vi "DAQ module.vi"(8 "error in (no error)":errorcluster) -> (0 "error out":errorcluster)   [LabVIEW 2016]
uses:
  Controls/Gain modes.ctl
  General/Controls/Queue modes.ctl
  General/Controls/staus modes.ctl
  General/Controls/DAQ device list.ctl
  General/Controls/data modes.ctl
  <vilib>/DAQmx/read.llb/DAQmx Read (Analog DBL 1Chan 1Samp).vi
  <vilib>/DAQmx/miscellaneous.llb/DAQmx Fill In Error Info.vi
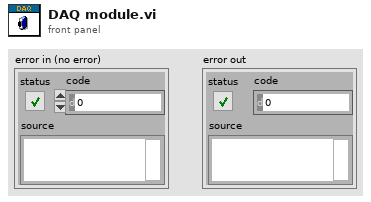
[diagram p1: front panel]
types:
  T1 = cluster{"seconds since 1Jan1904":timestamp, "Numeric 2":dbl}[]
  T2 = typedef "Queue modes.ctl" = enum16{"Initialise", "Destroy", "Get"}
  T3 = typedef "Gain modes.ctl" = enum16{"Initalise", "Get", "Set"}
  T4 = typedef "References.ctl" = cluster{"Tab Control":refnum<vi>, "Logo 1":refnum<vi>, "Logo 2":refnum<vi>, "Connect Actuator":refnum<vi>, "LIVE DATA":refnum<vi>, "Speed":refnum<vi>, "Home position":refnum<vi>, "Limit position":refnum<vi>, "Trigger":refnum<vi>, "Current position":refnum<vi>, "Connect Camera":refnum<vi>, "TEST DATA":refnum<vi>, "LIVE DATA Force":refnum<vi>, "Connect DAQ":refnum<vi>, "Initialised":refnum<vi>, "Test":refnum<vi>}
  T5 = typedef "staus modes.ctl" = enum16{"Status", "Testing", "Webcam", "DAQ", "Actuator", "Initialise"}
  T6 = typedef "DAQ device list.ctl" = enum16{"USB-6211", "NI myDAQ", "NI 9211"}
  T7 = typedef "data modes.ctl" = enum16{"Initalise", "Status", "Process", "Add load", "Add position"}
  T8 = enum16{"open", "replace", "create", "open or create", "replace or create", "replace or create with confirmation"}
  T9 = cluster{"seconds since 1Jan1904":timestamp, "data":dbl}[]
  T10 = typedef "DAQ queue.ctl" = cluster{"Sate":T11, "Data":variant}
  T11 = typedef "Queue states.ctl" = enum16{"Shutdown", "Save data", "Record", "Read", "Setup", "Zero", "Connect", "Initialise"}
  T12 = typedef "UEs.ctl" = cluster{"Read position":refnum<user-event>, "Check home":refnum<user-event>, "Record":refnum<user-event>, "Abort controller":refnum<user-event>, "Remote test":refnum<user-event>, "Test setup":refnum<user-event>, "Conditional wait":refnum<user-event>, "Abort move":refnum<user-event>, "Wait done":refnum<user-event>, "Send trigger":refnum<user-event>, "Initalising":refnum<user-event>, "Initalisation complete":refnum<user-event>}
  T13 = cluster{"seconds since 1Jan1904":timestamp, "Numeric":dbl}
  T14 = cluster{"seconds since 1Jan1904":timestamp, "Numeric":dbl}[]
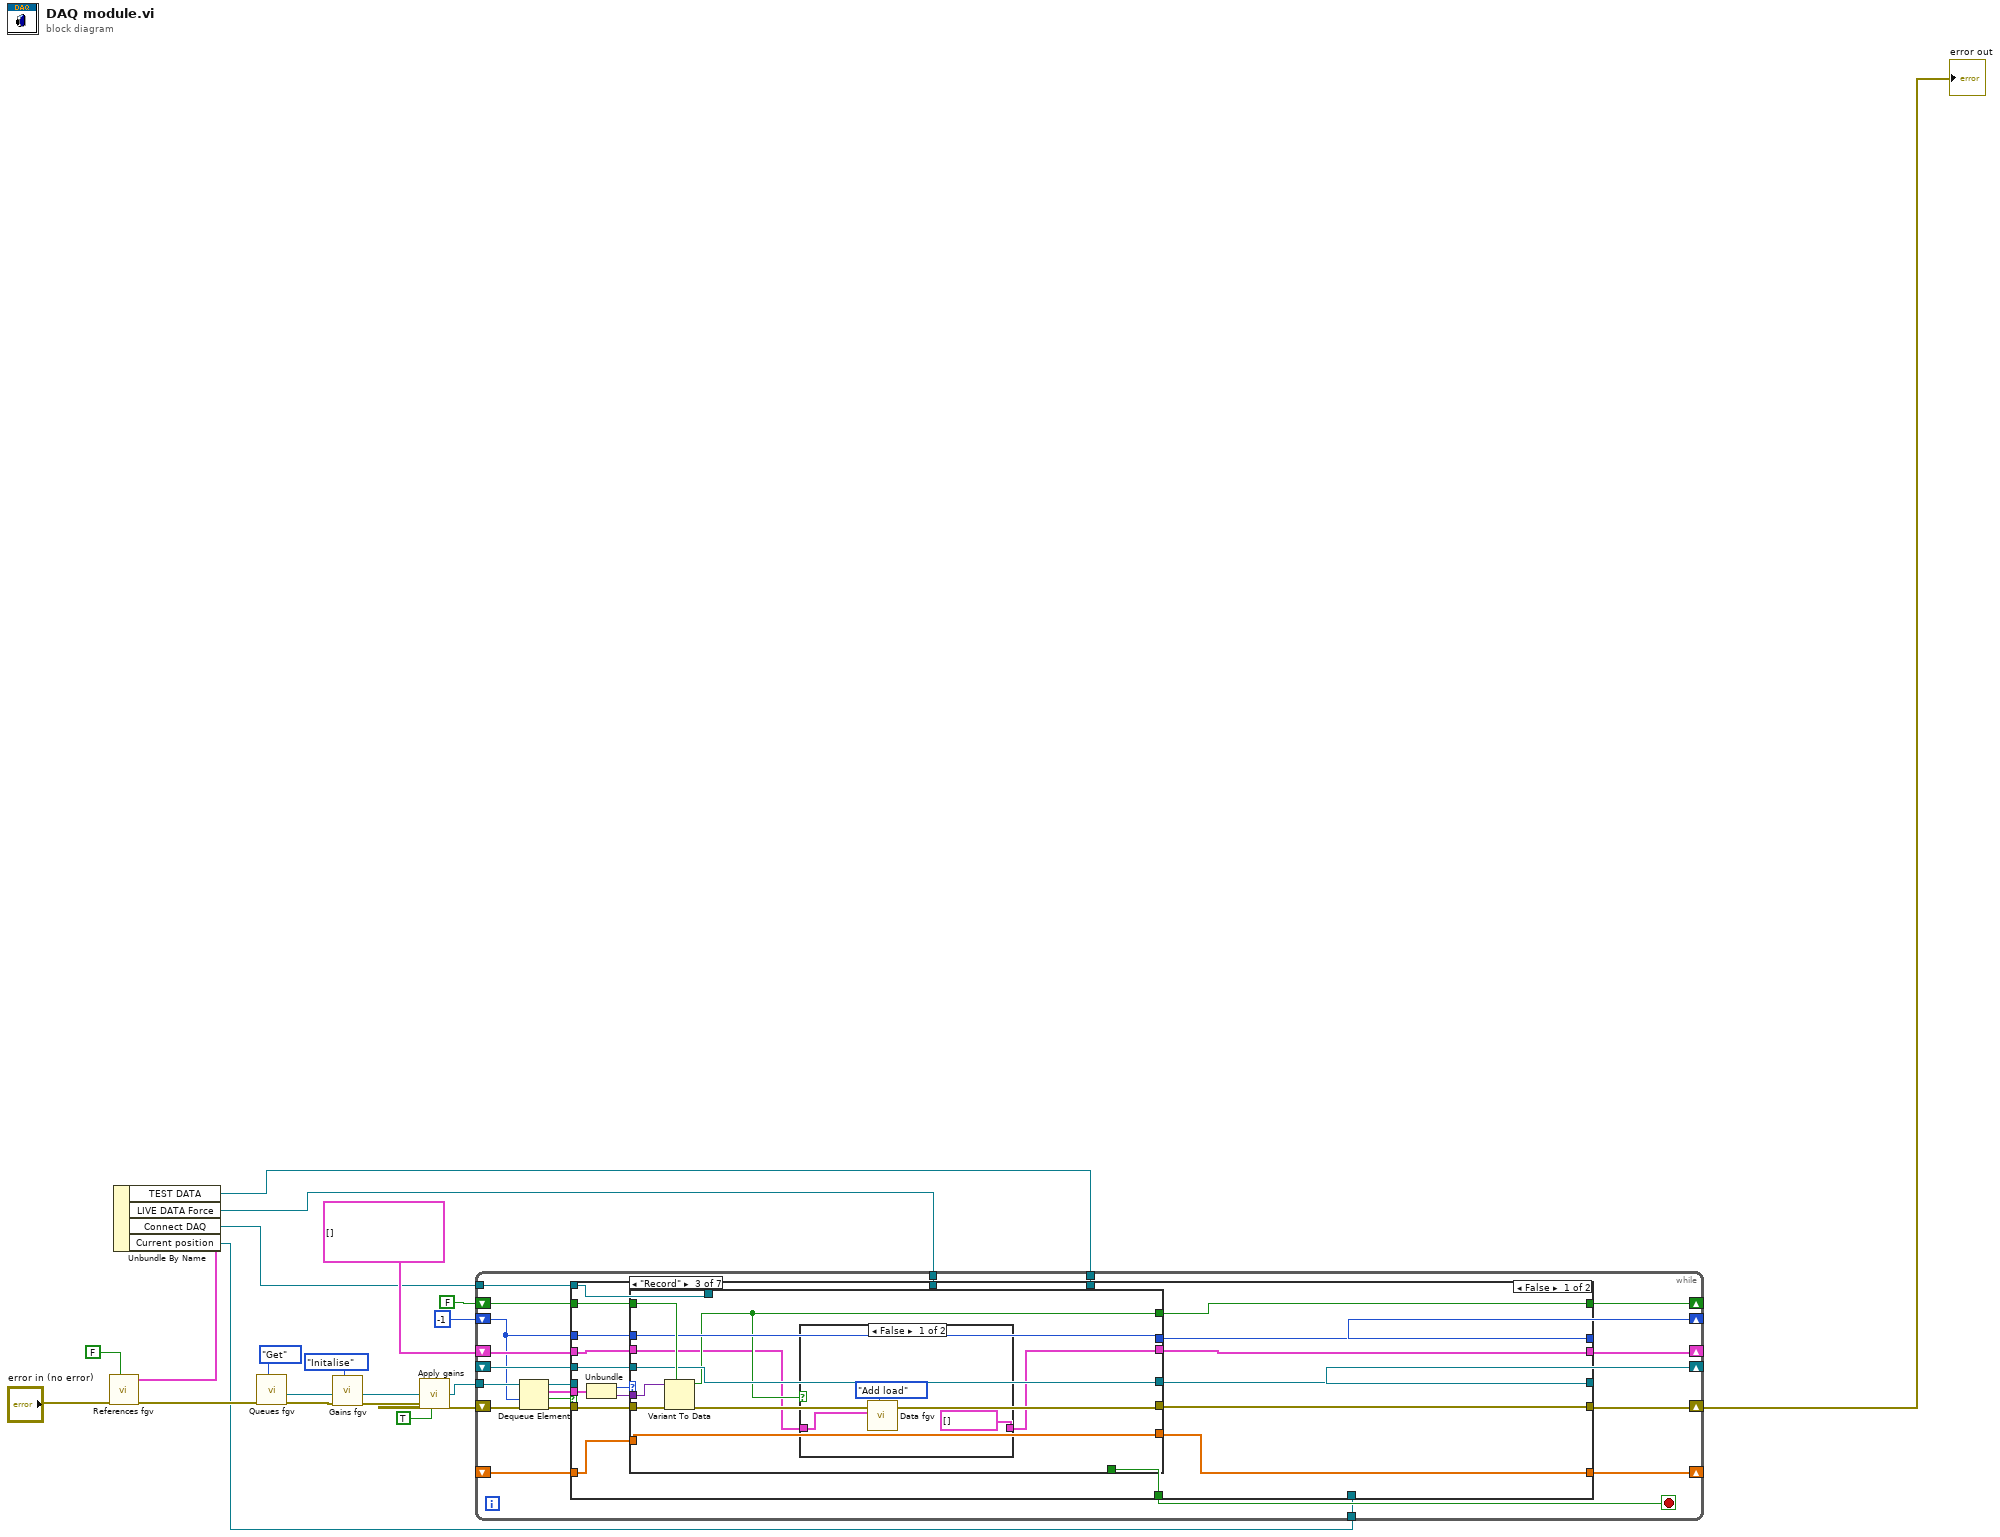
[diagram p0: block diagram]
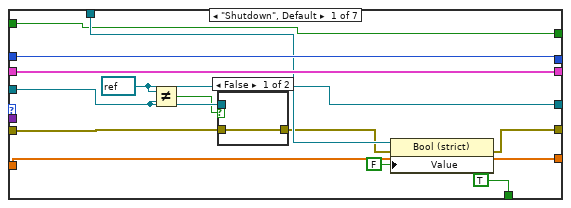
[diagram p2: hidden frame]
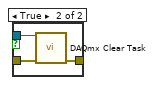
[diagram p3: hidden frame]
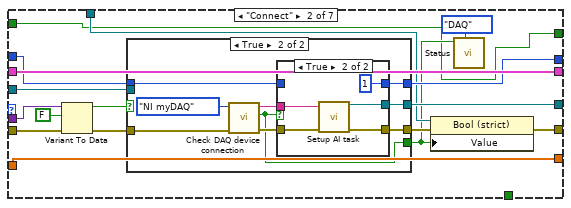
[diagram p4: hidden frame]
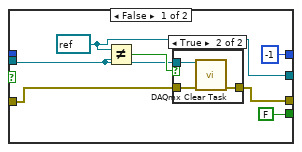
[diagram p5: hidden frame]
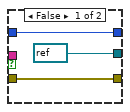
[diagram p7: hidden frame]
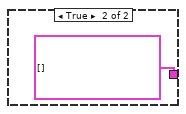
[diagram p8: hidden frame]
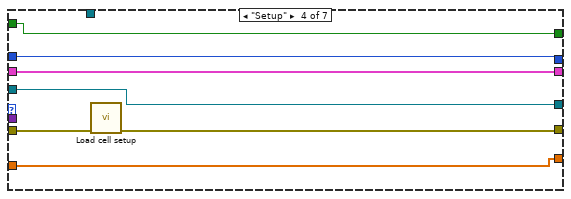
[diagram p9: hidden frame]
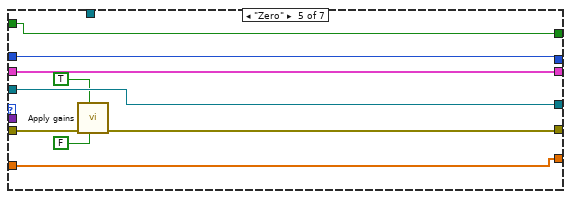
[diagram p10: hidden frame]
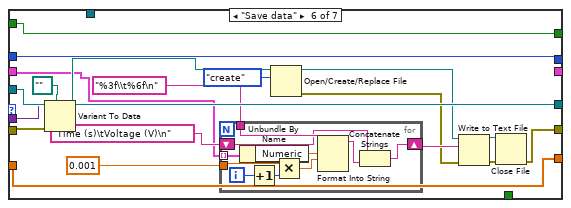
[diagram p11: hidden frame]
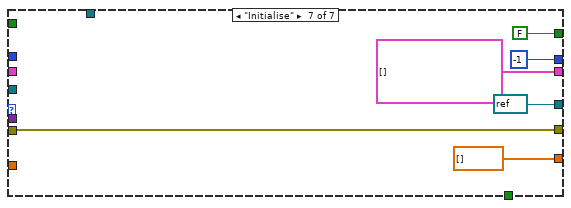
[diagram p12: hidden frame]
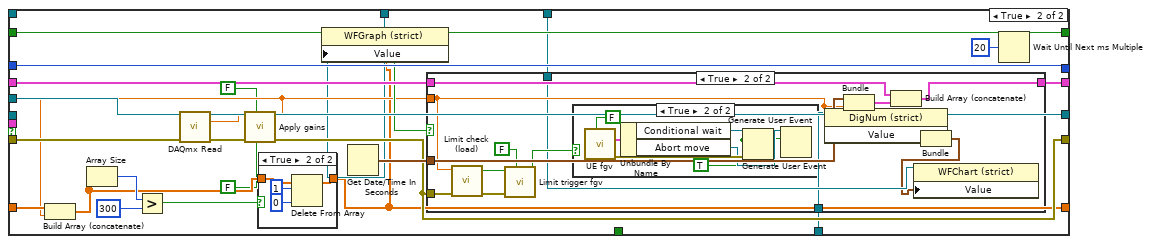
[diagram p13: hidden frame]
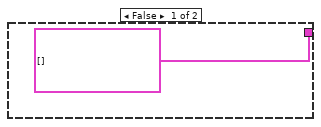
[diagram p14: hidden frame]
diagram:
  n1 = call "References fgv.vi"("Set?"=FALSE, "error in (no error)"="error in (no error)") -> ("error out"=w8:errorcluster, "Cluster"=w5:T4)  [unwired: 8 in]
  n2 = Unbundle By Name(w5) -> ("TEST DATA"=w2:refnum<vi>, "LIVE DATA Force"=w3:refnum<vi>, "Connect DAQ"=w4:refnum<vi>, "Current position"=w1:refnum<vi>)
  n3 = call "Queues fgv.vi"("Modes"=Queue_modes."Get", "error in (no error)"=w8) -> ("error in (no error) 2"=w18:errorcluster, "DAQ"=w17:refnum<queue>)  [unwired: 6 in, 2 out]
  n4 = call "Gains fgv.vi"("Mode"=Gain_modes."Initalise", "error in (no error)"=w18) -> ("error out"=w14:errorcluster)  [unwired: 7 in, 2 out]
  n5 = call "Apply gains.vi"("Initalise"=TRUE, "error in (no error)"=w14) -> ("error out"=w12:errorcluster)  [unwired: 8 in, 1 out]
  n6 = while {
    shift-right: [w40] -> _
    shift-left: _ -> [w41]
    shift-right: [w39] -> w10
    shift-left: w12 -> [w33]
    shift-right: [w38] -> _
    shift-left: T1 [] -> [w37]
    tunnel: w17 -> [w36]
    shift-right: [w29] -> _
    shift-left: -1 ("timeout in ms (-1)") -> [w30]
    tunnel: w4 -> [w28]
    shift-right: [w26] -> _
    shift-left: FALSE -> [w27]
    shift-right: [w23] -> _
    shift-left: _ -> [w24]
    tunnel: w3 -> [w22]
    tunnel: w2 -> [w21]
    tunnel: w1 -> [w20]
    stop <- w25 stop-if-true
    n7 = Dequeue Element(queue=w36, timeout in ms (-1)=w30, error in (no error)=w33) -> (queue out=w35:refnum<queue>, element=w31:T10, timed out?=w32:bool, error out=w34:errorcluster)
    n8 = case shown="False" w32 {
      tunnel: w41 -> [w50 w209]
      tunnel: w34 -> [w55 w203]
      tunnel: [w53 w208] -> w40
      tunnel: [w54 w190] -> w39
      tunnel: [w51 w207] -> w38
      tunnel: w37 -> [w52 w206]
      tunnel: w35 -> [_ _]
      tunnel: w31 -> [w58 _]
      tunnel: w30 -> [w49 w205]
      tunnel: [w48 w205] -> w29
      tunnel: w28 -> [w47 _]
      tunnel: w27 -> [w46 w204]
      tunnel: [w45 w204] -> w26
      tunnel: [w44 _] -> w25
      tunnel: w24 -> [w42 w200]
      tunnel: [w43 w188] -> w23
      tunnel: w22 -> [_ w189]
      tunnel: w21 -> [_ w187]
      tunnel: w20 -> [_ w186]
      frame False {
        n9 = Unbundle(w58) -> ("Sate"=w57:T11, "Data"=w56:variant)
        n10 = case shown="\"Record\"" w57 {
          tunnel: w56 -> [_ w87 w129 _ _ w164 _]
          tunnel: w55 -> [w70 w88 w130 w138 w145 w166 w183]
          tunnel: [w62 w81 w127 w137 w144 w153 w183] -> w54
          tunnel: [w69 w92 w126 w136 w147 w167 refnum<k21> refnum ("task out")] -> w53
          tunnel: w52 -> [w71 w91 w123 w139 w148 w152 _]
          tunnel: [w71 w91 w122 w139 w148 _ T9 []] -> w51
          tunnel: w50 -> [w68 w83 w126 w136 w147 w167 _]
          tunnel: w49 -> [w66 w90 w125 w140 w149 w169 _]
          tunnel: [w66 w89 w125 w140 w149 w169 -1 ("timeout in ms (-1)")] -> w48
          tunnel: w47 -> [w65 w80 _ _ _ _ _]
          tunnel: w46 -> [w61 w77 w128 w141 w150 w168 _]
          tunnel: [w61 w77 w124 w141 w150 w168 FALSE] -> w45
          tunnel: [TRUE _ _ _ _ _ _] -> w44
          tunnel: [w59 w76 w121 w135 w146 w151 dbl[] []] -> w43
          tunnel: w42 -> [w59 w76 w121 w135 w146 w151 _]
          frame "Shutdown", Default {
            w69 = refnum<k21> refnum ("task out")
            n11 = Not Equal?(x=w69, y=w68) -> (x != y?=w67:bool)
            n12 = case shown="False" w67 {
              tunnel: w70 -> [w72 w75]
              tunnel: [w72 w74] -> w63
              tunnel: w68 -> [_ w73]
              frame False {
              }
              frame True {
                n13 = call <vilib>:"DAQmx Clear Task.vi"("task in"=w73, "error in"=w75) -> ("error out"=w74:errorcluster)  [unwired: 13 in]
              }
            }
            n14 = property class="Bool (strict)"(reference=w65, error in=w63, "Value"=FALSE) -> (error out=w62:errorcluster)  [unwired: 1 out]
          }
          frame "Connect" {
            n15 = Variant To Data(error in=w88, type=FALSE, Variant=w87) -> (data=w84:bool, error out=w86:errorcluster)
            n16 = case shown="True" w84 {
              tunnel: [w95 w109] -> w82
              tunnel: [w97 w108] -> w92
              tunnel: w90 -> [_ w107]
              tunnel: [-1 ("timeout in ms (-1)") w106] -> w89
              tunnel: w86 -> [w94 w105]
              tunnel: w83 -> [w98 _]
              tunnel: [FALSE ("x != y?") w104] -> w78
              frame False {
                w97 = refnum<k21> refnum ("task out")
                n17 = Not Equal?(x=w97, y=w98) -> (x != y?=w99:bool)
                n18 = case shown="True" w99 {
                  tunnel: w94 -> [w100 w103]
                  tunnel: [w100 w102] -> w95
                  tunnel: w98 -> [_ w101]
                  frame False {
                  }
                  frame True {
                    n19 = call <vilib>:"DAQmx Clear Task.vi"("task in"=w101, "error in"=w103) -> ("error out"=w102:errorcluster)  [unwired: 13 in]
                  }
                }
              }
              frame True {
                n20 = call "Check DAQ device connection.vi"("error in (no error)"=w105, "DAQ Device"=DAQ_device_list."NI myDAQ") -> ("error out"=w111:errorcluster, "Device Present?"=w104:bool, "DAQmx Device Name"=w112:tag)  [unwired: 7 in]
                n21 = case shown="True" w104 {
                  tunnel: w111 -> [w114 w120]
                  tunnel: w112 -> [_ w119]
                  tunnel: [refnum<k21> refnum ("task out") w118] -> w108
                  tunnel: [w114 w117] -> w109
                  tunnel: w107 -> [w113 _]
                  tunnel: [w113 1 ("timeout in ms (-1)")] -> w106
                  frame False {
                  }
                  frame True {
                    n22 = call "Setup AI task.vi"("error in"=w120, "DAQmx Device Name"=w119) -> ("error out"=w117:errorcluster, "task out"=w118:refnum<k21>)  [unwired: 8 in]
                  }
                }
              }
            }
            n23 = property class="Bool (strict)"(reference=w80, error in=w82, "Value"=w78) -> (error out=w81:errorcluster)  [unwired: 1 out]
            n24 = call "Status.vi"("Mode"=staus_modes."DAQ", "Data"=w78) -> ()  [unwired: 7 in, 3 out]
          }
          frame "Record" {
            n25 = Variant To Data(error in=w130, type=w128, Variant=w129) -> (data=w124:bool, error out=w127:errorcluster)
            n26 = case shown="False" w124 {
              tunnel: w123 -> [w131 _]
              tunnel: [T1 [] T1 []] -> w122
              frame False {
                n27 = call "Data fgv.vi"("Modes"=data_modes."Add load", "Data"=w131) -> ()  [unwired: 5 in, 5 out]
              }
              frame True {
              }
            }
          }
          frame "Setup" {
            n28 = call "Load cell setup.vi"("error in (no error)"=w138) -> ("error out"=w137:errorcluster)  [unwired: 10 in]
          }
          frame "Zero" {
            n29 = call "Apply gains.vi"("Initalise"=FALSE, "Zero?"=TRUE, "error in (no error)"=w145) -> ("error out"=w144:errorcluster)  [unwired: 7 in, 1 out]
          }
          frame "Save data" {
            n30 = Variant To Data(error in=w166, type=path "" ("file path (dialog if empty)"), Variant=w164) -> (data=w160:path)  [unwired: 1 out]
            n31 = for {
              tunnel: w152 -> [w171] mode=indexing
              tunnel: 0.001 ("dt") -> [w179]
              tunnel: "%3f\\t%6f\n" ("format string") -> [w176]
              shift-right: [w173] -> w157
              shift-left: "Time (s)\tVoltage (V)\n" ("format string") -> [w174]
              i -> [w178]
              n32 = Unbundle By Name(w171) -> ("Numeric"=w170:dbl)
              n33 = Increment(x=w178) -> (x+1=w177:i32)
              n34 = Multiply(x=w179, y=w177) -> (x*y=w172:dbl)
              n35 = Format Into String(format string=w176, w172, w170) -> (resulting string=w175:string)  [unwired: 2 in, 1 out]
              n36 = Concatenate Strings(w174, w175) -> (w173:string)
            }
            n37 = Open/Create/Replace File(file path (use dialog)=w160, operation (0:open)=T8."create") -> (refnum out=w158:refnum<file>, error out=w156:errorcluster)  [unwired: 4 in, 1 out]
            n38 = Write to Text File(file (use dialog)=w158, text=w157, error in=w156) -> (refnum out=w154:refnum<file>, error out=w155:errorcluster)  [unwired: 1 in, 1 out]
            n39 = Close File(refnum=w154, error in=w155) -> (error out=w153:errorcluster)  [unwired: 1 out]
          }
          frame "Initialise" {
          }
        }
      }
      frame True {
        n40 = call-poly <vilib>:"DAQmx Read.vi"("task/channels in"=w209, "error in"=w203) -> ("task out"=w208:refnum<k21>, "data"=w192:dbl, "error out"=w191:errorcluster)  [unwired: 11 in]
        n41 = call "Apply gains.vi"("Initalise"=FALSE, "Zero?"=FALSE, "error in (no error)"=w191, "Voltage"=w192) -> ("error out"=w190:errorcluster, "Numeric"=w195:dbl)  [unwired: 6 in]
        n42 = Build Array (concatenate)(w200, w195) -> (w197:dbl[])
        n43 = Array Size(array=w197) -> (size(s)=w199:i32)
        n44 = Greater?(x=w199, y=300) -> (0:w196:bool)
        n45 = case shown="True" w196 {
          tunnel: w197 -> [w231 w235]
          tunnel: [w231 w232] -> w188
          frame False {
          }
          frame True {
            n46 = Delete From Array(array=w235, length=1, index=0) -> (array with subset deleted=w232:dbl[])  [unwired: 1 out]
          }
        }
        n47 = property class="WFGraph (strict)"(reference=w189, "Value"=w188) -> ()  [unwired: 1 in, 2 out]
        n48 = Get Date/Time In Seconds() -> (seconds since 1Jan1904=w202:timestamp)
        n49 = case shown="True" w204 {
          tunnel: w195 -> [_ w219]
          tunnel: [T9 [] w221] -> w207
          tunnel: w206 -> [_ w223]
          tunnel: w202 -> [_ w224]
          tunnel: w190 -> [_ w214]
          tunnel: w187 -> [_ w213]
          tunnel: w186 -> [_ w211]
          frame False {
          }
          frame True {
            n50 = call "Limit check (load).vi"("error in (no error)"=w214, "Load"=w219) -> ("error out"=w217:errorcluster, "Limit?"=w216:bool)  [unwired: 8 in]
            n51 = call "Limit trigger fgv.vi"("Reset"=FALSE, "error in (no error)"=w217, "Set"=w216) -> ("Limit trigger"=w218:bool)  [unwired: 7 in, 1 out]
            n52 = case shown="True" w218 {
              frame False {
              }
              frame True {
                w225 = TRUE ("event data")
                n53 = call "UE fgv.vi"("Set?"=FALSE) -> ("error out"=w229:errorcluster, "UEs"=w230:T12)  [unwired: 8 in, 1 out]
                n54 = Unbundle By Name(w230) -> ("Conditional wait"=w227:refnum<user-event>, "Abort move"=w226:refnum<user-event>)
                n55 = Generate User Event(user event=w227, event data cluster=w225, error in=w229) -> ()  [unwired: 1 in, 2 out]
                n56 = Generate User Event(user event=w226, event data cluster=w225) -> ()  [unwired: 2 in, 2 out]
              }
            }
            n57 = property on="Property Node" class="DigNum (strict)"(reference=w211) -> ("Value"=w220:dbl)  [unwired: 1 in, 2 out]
            n58 = Bundle("seconds since 1Jan1904"=w224, "Numeric"=w219) -> (w222:T13)  [unwired: 1 in]
            n59 = Build Array (concatenate)(w223, w222) -> (w221:T14)
            n60 = Bundle("Value"=w220, "Numeric"=w219) -> (w212:cluster{"Value":dbl, "Numeric":dbl})  [unwired: 1 in]
            n61 = property class="WFChart (strict)"(reference=w213, "Value"=w212) -> ()  [unwired: 1 in, 2 out]
          }
        }
        n62 = Wait Until Next ms Multiple(millisecond multiple=u32 20) -> ()  [unwired: 1 out]
      }
    }
  }
  "error out" <- w10
